vi "check change (SubVI).vi"(11 "Array in":T1(array[cluster])) -> (3 "Array out":bool[](array[boolean]))   [LabVIEW 2016]
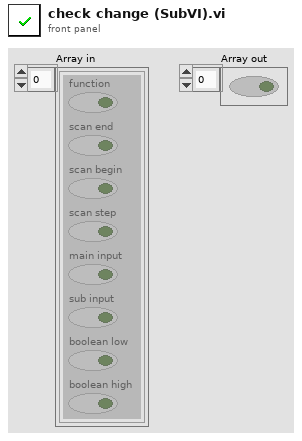
[diagram p1: front panel]
types:
  T1 = cluster{"function":bool, "scan end":bool, "scan begin":bool, "scan step":bool, "main input":bool, "sub input":bool, "boolean low":bool, "boolean high":bool}[]
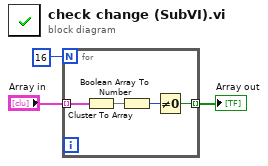
[diagram p0: block diagram]
diagram:
  n1 = for {
    N: 16 -> [_]
    tunnel: "Array in" -> [w5] mode=indexing
    tunnel: [w4] -> w3 mode=indexing
    n2 = Cluster To Array(cluster=w5) -> (array=w6:bool[])
    n3 = Boolean Array To Number(Boolean array=w6) -> (number=w7:u32)
    n4 = Not Equal To 0?(x=w7) -> (x != 0?=w4:bool)
  }
  "Array out" <- w3
